vi "Query Self-Alignment Last Status.vi"(8 "error in (no error)":errorcluster, 11 "VISA resource name":refnum<visa-resource-name>) -> (0 "error out":errorcluster, 1 "StateLevel":i32, 2 "StateIQ":i32, 3 "VISA resource name out":refnum<visa-resource-name>)   [LabVIEW 2015, in "Rohde&Schwarz CMXP Base.lvlib"]
doc: "Queries status information for the last self-alignment execution. The information is returned for the measurement modes \"IQ\" or \"Verify IQ\" (whichever was executed last) and \"Level\":\n\nAttribute:\nRSCMXPBASE_ATTR_QUERY_LAST_MEASURMENT_MODE\n\nRemote-control command:\nFETCh:BASE:SALignment:STATe?"
uses:
  <instrlib>/Rohde&Schwarz CMXP Base/Rohde&Schwarz CMXP Base.lvlib
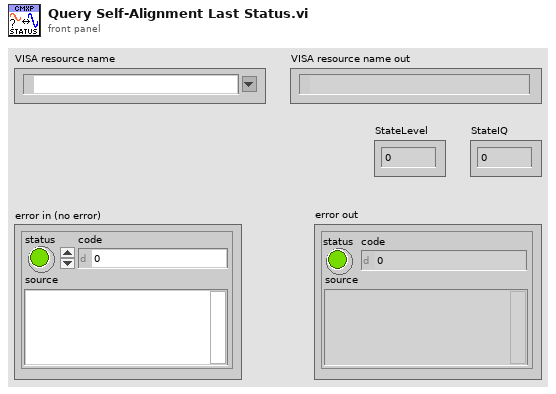
[diagram p1: front panel]
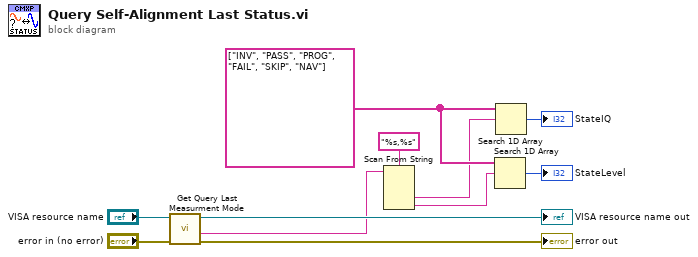
[diagram p0: block diagram]
diagram:
  w4 = string[] ["INV", "PASS", "PROG", "FAIL", "SKIP", "NAV"]
  n1 = call "Get Query Last Measurment Mode"("error in (no error)"="error in (no error)", "instrument handle"="VISA resource name") -> ("error out"=→"error out":errorcluster, "Query Last Measurment Mode"=w1:string, "instrument handle out"=→"VISA resource name out":refnum<visa-resource-name>)  [unwired: 7 in]
  n2 = Scan From String(format string="%s,%s", input string=w1) -> (output 1=w3:string, output 2=w2:string)  [unwired: 4 in, 3 out]
  n3 = Search 1D Array(1D array=w4, element=w2) -> (index of element=→"StateLevel":i32)  [unwired: 1 in]
  n4 = Search 1D Array(1D array=w4, element=w3) -> (index of element=→"StateIQ":i32)  [unwired: 1 in]
